vi "tutorial-062.vi"() -> ()   [LabVIEW 2019]
uses:
  TextControlledInstrum/TextControlledInstrum.lvlib
  TextControlledInstrum/IOQueuePacket.ctl
  TextControlledInstrum/ControlToCommandMulti.vi
panel:
  in  "B Delay (s)":dbl format="%#_6p"
  in  "B Origin":T1(ring)
  in  "B DLAY":string="LAMP 1,%g\nLAMP? 1\n%g\nLOFF 1,%g\nLOFF? 1\n%g\nLPOL 1,%d\nLPOL? 1\n%d\n"
  in  "A Delay (s)":dbl format="%#_6p"
  in  "A Origin":T1(ring)
  in  "A DLAY":string="LAMP 1,%g\nLAMP? 1\n%g\nLOFF 1,%g\nLOFF? 1\n%g\nLPOL 1,%d\nLPOL? 1\n%d\n"
  in  "AB Polarity":enum16{"Neg", "Pos"}(ring)
  in  "AB Offset (V)":dbl
  in  "VISA resource name":refnum<visa-resource-name>
  in  "AB Amplitude (V)":dbl
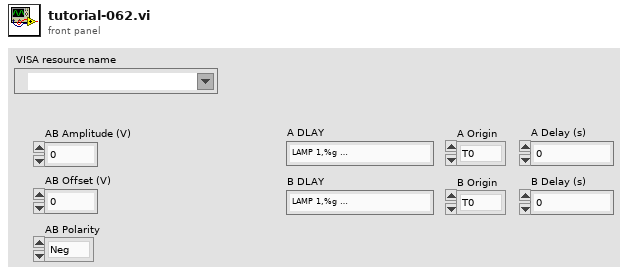
[diagram p1: front panel]
types:
  T1 = enum16{"T0", "T1", "A", "B", "C", "D", "E", "F", "G", "H"}
  T2 = typedef "TextControlledInstrum.lvlib/IOQueuePacket.ctl" = cluster{"Operation":enum16{"read", "write", "reserved2", "reserved3", "reserved4", "reserved5", "reserved6", "reserved7"}, "Data":string, "Queue":refnum<queue>}
  T3 = enum16{"read", "write", "reserved2", "reserved3", "reserved4", "reserved5", "reserved6", "reserved7"}
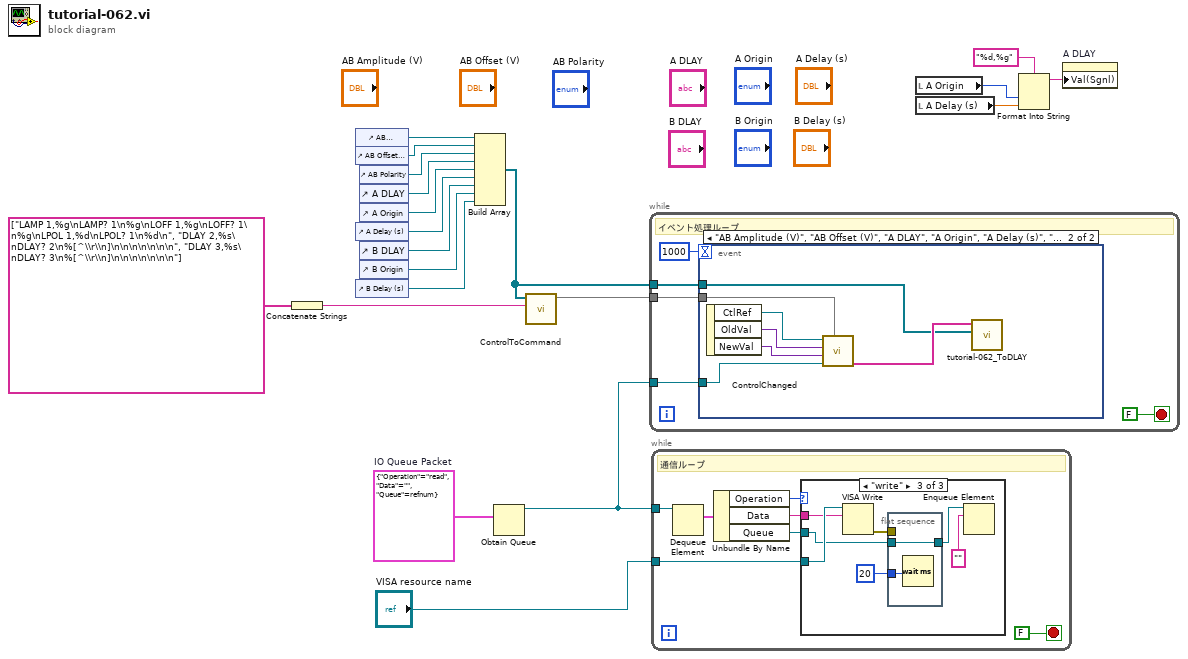
[diagram p0: block diagram]
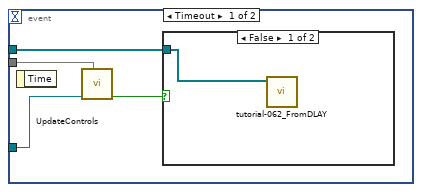
[diagram p2: hidden frame]
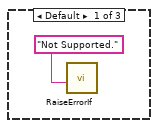
[diagram p4: hidden frame]
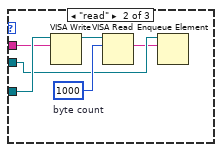
[diagram p5: hidden frame]
diagram:
  w18 = T2 {"Operation"=enum."read", "Data"="", "Queue"=refnum}  # IO Queue Packet
  n1 = Concatenate Strings(string[] ["LAMP 1,%g\nLAMP? 1\n%g\nLOFF 1,%g\nLOFF? 1\n%g\nLPOL 1,%d\nLPOL? 1\n%d\n", "DLAY 2,%s\nDLAY? 2\n%[^\\r\\n]\n\n\n\n\n\n\n", "DLAY 3,%s\nDLAY? 3\n%[^\\r\\n]\n\n\n\n\n\n\n"]) -> (w6:string)
  n2 = control-ref of="AB Amplitude (V)"() -> (w20:refnum<vi>)
  n3 = control-ref of="AB Offset (V)"() -> (w15:refnum<vi>)
  n4 = control-ref of="A Delay (s)"() -> (w11:refnum<vi>)
  n5 = control-ref of="B Delay (s)"() -> (w9:refnum<vi>)
  n6 = control-ref of="AB Polarity"() -> (w14:refnum<vi>)
  n7 = control-ref of="A DLAY"() -> (w13:refnum<vi>)
  n8 = control-ref of="A Origin"() -> (w12:refnum<vi>)
  n9 = control-ref of="B DLAY"() -> (w10:refnum<vi>)
  n10 = control-ref of="B Origin"() -> (w8:refnum<vi>)
  n11 = Build Array(w20, w15, w14, w13, w12, w11, w10, w8, w9) -> (w5:refnum<vi>[])
  n12 = Obtain Queue(element data type=w18) -> (queue out=w16:refnum<queue>)  [unwired: 4 in, 2 out]
  n13 = call-poly "ControlToCommand.vi"("SetGetCommands"=w6, "Control Array"=w5) -> ("ControlToCommand"=w19:map{refnum<vi>, string[]})  [unwired: 9 in]
  n14 = while {
    tunnel: w19 -> [w25]
    tunnel: w16 -> [w24]
    tunnel: w5 -> [w21]
    stop <- FALSE stop-if-true
    # "イベント処理ループ"
    n15 = event shown="[1] \"AB Amplitude (V)\", \"AB Offset (V)\", \"A DLAY\", \"A Origin\", \"A Delay (s)\", \"B DLAY\", \"B Origin\", \"B Delay (s)\": Value Change" {
      selector: _ -> [_ _]
      dyn-events: _ -> [_ _]
      timeout: 1000 -> [_ _]
      tunnel: w25 -> [w29 w37]
      tunnel: w24 -> [w28 w33]
      tunnel: w21 -> [w26 w31]
      event Timeout {
        n16 = event-data() -> ()  [unwired: 1 in, 1 out]
        n17 = call "UpdateControls.vi"("ControlToCommand"=w29, "IO Queue"=w28) -> ("timed out?"=w27:bool)  [unwired: 9 in]
        n18 = case shown="False" w27 {
          tunnel: w26 -> [w30 _]
          frame False {
            n19 = call "tutorial-062_FromDLAY.vi"("Control Array"=w30) -> ()  [unwired: 11 in]
          }
          frame True {
          }
        }
      }
      event "AB Amplitude (V)", "AB Offset (V)", "A DLAY", "A Origin", "A Delay (s)", "B DLAY", "B Origin", "B Delay (s)": Value Change {
        n20 = event-data() -> ("CtlRef"=w36:refnum<vi>, "OldVal"=w35:variant, "NewVal"=w34:variant)  [unwired: 1 in]
        n21 = call "ControlChanged.vi"("ControlToCommand"=w37, "IO Queue"=w33, "NewVal"=w34, "OldVal"=w35, "CtlRef"=w36) -> ("Changed Names out"=w32:string[])  [unwired: 6 in]
        n22 = call "tutorial-062_ToDLAY.vi"("Control Array"=w31, "Changed Names"=w32) -> ()  [unwired: 10 in]
      }
    }
  }
  n23 = while {
    tunnel: w16 -> [w44]
    tunnel: "VISA resource name" -> [w41]
    stop <- FALSE stop-if-true
    # "通信ループ"
    n24 = Dequeue Element(queue=w44) -> (element=w43:T2)  [unwired: 2 in, 3 out]
    n25 = Unbundle By Name(w43) -> ("Operation"=w42:T3, "Data"=w40:string, "Queue"=w39:refnum<queue>)
    n26 = case shown="\"write\"" w42 {
      tunnel: w41 -> [_ w49 w58]
      tunnel: w40 -> [_ w48 w57]
      tunnel: w39 -> [_ w47 w55]
      frame Default {
        n27 = call "RaiseErrorIf.vi"("error message"="Not Supported.") -> ()  [unwired: 10 in, 1 out]
      }
      frame "read" {
        w50 = u32 1000  # byte count
        n28 = VISA Write(VISA resource name=w49, write buffer=w48) -> (VISA resource name out=w51:refnum<visa-resource-name>)  [unwired: 1 in, 2 out]
        n29 = VISA Read(VISA resource name=w51, byte count=w50) -> (read buffer=w46:string)  [unwired: 1 in, 3 out]
        n30 = Enqueue Element(queue=w47, element=w46) -> ()  [unwired: 2 in, 3 out]
      }
      frame "write" {
        n31 = VISA Write(VISA resource name=w58, write buffer=w57) -> (error out=w53:errorcluster)  [unwired: 1 in, 2 out]
        n32 = flat-sequence {
          tunnel: u32 20 ("milliseconds to wait") -> [w61]
          tunnel: w55 -> [w60]
          tunnel: [w60] -> w54
          tunnel: [w59] -> _
          tunnel: w53 -> [w59]
          frame #0 {
            n33 = Wait (ms)(milliseconds to wait=w61) -> ()  [unwired: 1 out]
          }
        }
        n34 = Enqueue Element(queue=w54, element="") -> ()  [unwired: 2 in, 3 out]
      }
    }
  }
  n35 = local read "A Origin"() -> (w4:T1)
  n36 = local read "A Delay (s)"() -> (w3:dbl)
  n37 = Format Into String(format string="%d,%g", w4, w3) -> (resulting string=w2:string)  [unwired: 2 in, 1 out]
  n38 = property on="A DLAY" class="Str"("Val(Sgnl)"=w2) -> ()  [unwired: 2 in, 2 out]
